vi "NXTServo-DM.vi"(0 "Input of NXTServo":T1={"Servo Number"=1, "Position"=1500, "Speed"=0} {"Speed" step=1 scale=0.0..255.0; "Position" min=500 max=2500 step=1 scale=500.0..2500.0; "Servo Number" min=1 max=8 step=1}, 2 "NXT":T3={"Hardware"="NXT", "Flattened String"=""}, 3 "Input Port":T2 items=["Port 1", "Port 2", "Port 3", "Port 4"]) -> (1 "Output of NXTServo":cluster{"Voltage":u8, "Status":bool}, 4 "NXT dup":T3={"Hardware"="NXT", "Flattened String"=""} caption="NXT")   [LabVIEW 2012]
uses:
  <vilib>/NXT/Subs/LVHSConnector.ctl
  <vilib>/NXT/Block Support/NXT_InputPort.ctl
  <vilib>/NXT/Block Support/HWPage.SensorType.ctl
  <vilib>/NXT/Block Support/HWPage.SensorMode.ctl
panel:
  # "mindsensors.com\nCopyright (c) 2009 by mindsensors.com\nEmail: info (<at>) mindsensors (<dot>) com\n\nThis program is free software. You can redistribute it and/or modify\nit under the terms of the GNU General Public License as published by\nthe Free Software Foundation; version 3 of the License.\nRead the license at: http://www.gnu.org/licenses/gpl.txt"
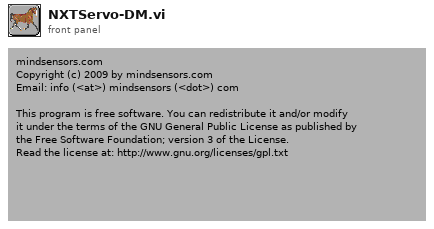
[diagram p1: front panel]
types:
  T1 = cluster{"Servo Number":u8, "Position":u16, "Speed":u8}
  T2 = typedef "NXT_InputPort.ctl" = u8
  T3 = typedef "LVHSConnector.ctl" = cluster{"Hardware":string, "Flattened String":string}
  T4 = typedef "HWPage.SensorType.ctl" = u8
  T5 = typedef "HWPage.SensorMode.ctl" = u8
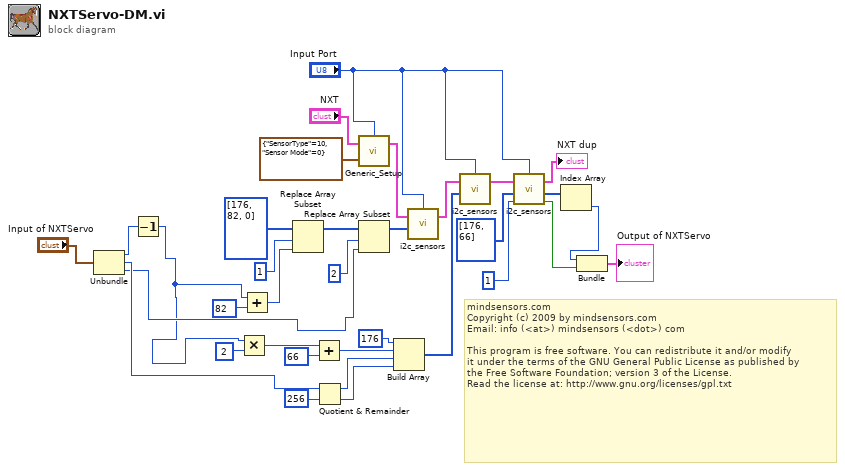
[diagram p0: block diagram]
diagram:
  # "mindsensors.com\nCopyright (c) 2009 by mindsensors.com\nEmail: info (<at>) mindsensors (<dot>) com\n\nThis program is free software. You can redistribute it and/or modify\nit under the terms of the GNU General Public License as published by\nthe Free Software Foundation; version 3 of the License.\nRead the license at: http://www.gnu.org/licenses/gpl.txt"
  n1 = Unbundle("Input of NXTServo") -> ("Servo Number"=w2:u8, "Position"=w7:u16, "Speed"=w6:u8)
  n2 = Decrement(x=w2) -> (x-1=w1:u8)
  n3 = Multiply(x=w1, y=u8 2) -> (x*y=w19:u8)
  n4 = Add(x=w1, y=u8 82 ("register")) -> (x+y=w31:u8)
  n5 = Replace Array Subset(array=i32[] [176, 82, 0] ("Commands"), new element=w31, index=1) -> (w30:i32[])
  n6 = Add(x=w19, y=u8 66 ("register")) -> (x+y=w15:u8)
  n7 = Quotient & Remainder(x=w7, y=u16 256) -> (x-y*floor(x/y)=w16:u16, floor(x/y)=w17:u16)
  n8 = call <vilib>:"Generic_Setup.vi"("Sensor Setup"=cluster{"SensorType":T4, "Sensor Mode":T5} {"SensorType"=10, "Sensor Mode"=0}, "NXT"="NXT", "Port"="Input Port") -> ("NXT"=w10:T3)  [unwired: 1 out]
  n9 = Replace Array Subset(array=w30, new element=w6, index=2) -> (w26:i32[])
  n10 = Build Array(u8 176 ("Device Address"), w15, w16, w17) -> (w13:u16[])
  n11 = call <vilib>:"i2c_sensors.vi"("Bytes to Write"=w26, "NXT"=w10, "Port"="Input Port") -> ("NXT"=w9:T3)  [unwired: 2 in, 2 out]
  n12 = call <vilib>:"i2c_sensors.vi"("Bytes to Write"=w13, "NXT"=w9, "Port"="Input Port") -> ("NXT"=w12:T3)  [unwired: 2 in, 2 out]
  n13 = call <vilib>:"i2c_sensors.vi"("Return Length"=1 ("LS Response Length (0)"), "Bytes to Write"=u8[] [176, 66] ("Buffer"), "NXT"=w12, "Port"="Input Port") -> ("Success?"=w4:bool, "Bytes read"=w23:u8[], "NXT"=→"NXT dup":T3)  [unwired: 1 in]
  n14 = Index Array(array=w23) -> (element=w5:u8)  [unwired: 1 in]
  n15 = Bundle(w5, "Success?"=w4) -> (→"Output of NXTServo":cluster{u8, "Success?":bool})  [unwired: 1 in]
